vi "formatIntoStringArray.vi"(8 "error in (no error)":errorcluster, 11 "Category in":refnum<class "Category.lvclass">) -> (0 "error out":errorcluster, 2 "2D Display":string[](array[string]), 3 "Category out":refnum<class "Category.lvclass">)   [LabVIEW 2018, in "Category.lvclass"]
uses:
  Category.lvclass
  Category.lvclass/Category.ctl
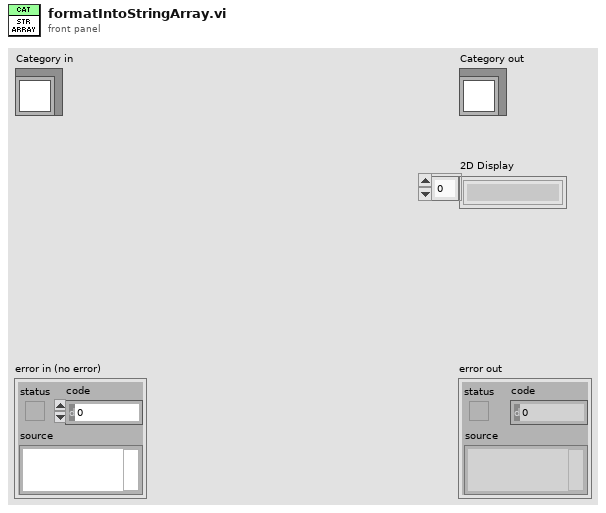
[diagram p1: front panel]
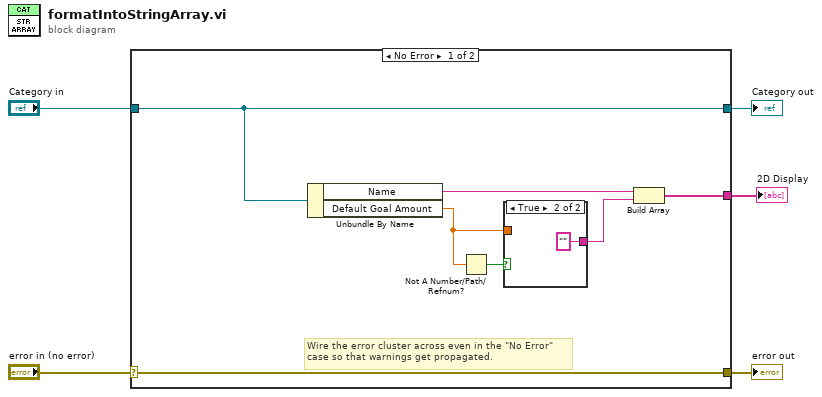
[diagram p0: block diagram]
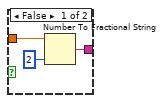
[diagram p2: hidden frame]
diagram:
  n1 = case shown="No Error" "error in (no error)" {
    selector: "error in (no error)" -> [w12 w18]
    tunnel: [w12 w18] -> w4
    tunnel: [w11 w17] -> w2
    tunnel: "Category in" -> [w11 w17]
    tunnel: [w8 _] -> w1
    frame No Error {
      # "Wire the error cluster across even in the \"No Error\"\ncase so that warnings get propagated."
      n2 = Unbundle By Name(w11) -> ("Name"=w10:string, "Default Goal Amount"=w7:dbl)
      n3 = Not A Number/Path/Refnum?(number/path/refnum=w7) -> (NaN/Path/Refnum?=w6:bool)
      n4 = case shown="True" w6 {
        tunnel: [w14 ""] -> w9
        tunnel: w7 -> [w13 _]
        frame False {
          n5 = Number To Fractional String(number=w13, precision (6)=i16 2) -> (F-format string=w14:string)  [unwired: 2 in]
        }
        frame True {
        }
      }
      n6 = Build Array(w10, w9) -> (w8:string[])
    }
    frame Error {
    }
  }
  "error out" <- w4
  "Category out" <- w2
  "2D Display" <- w1
